vi "Agilent ENA Series Short Calibration.vi"() -> ()   [LabVIEW 2020]
doc: "Performs short calibration for port 1 and port 2.\n\nFor this VI you must set SHORT Port 1 and Port 2 on instrument."
uses:
  <instrlib>/Agilent ENA Series/Agilent ENA Series.lvlib
panel:
  in  "Reset? (T: Yes)":bool=TRUE
  in  "ID Query? (T: Yes)":bool=TRUE
  in  "VISA resource name":refnum<visa-resource-name>
  # "(c) 2005-2021 National Instruments.  ALL RIGHTS RESERVED."
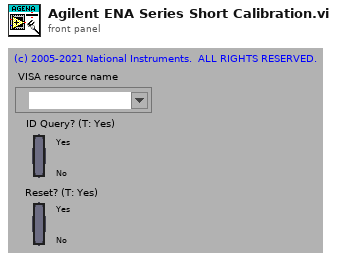
[diagram p1: front panel]
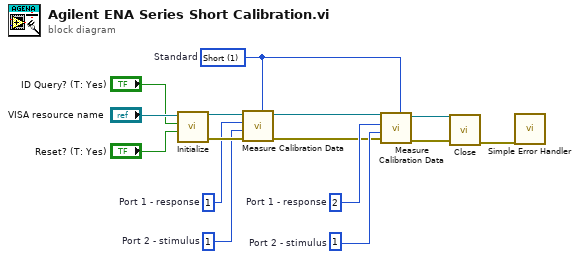
[diagram p0: block diagram]
diagram:
  w6 = 1  # Port 2 - stimulus
  w7 = 2  # Port 1 - response
  w9 = 1  # Port 2 - stimulus
  w10 = 1  # Port 1 - response
  w8 = u16 1 items=["Open", "Short", "Load", "Trhu", "Isolation"]  # Standard
  n1 = call <instrlib>:"Initialize.vi"("Reset? (T: Yes)"="Reset? (T: Yes)", "ID Query? (T: Yes)"="ID Query? (T: Yes)", "VISA resource name"="VISA resource name") -> ("error out"=w11:errorcluster, "VISA resource name out"=w12:refnum<visa-resource-name>)  [unwired: 7 in]
  n2 = call <instrlib>:"Measure Calibration Data.vi"("Standard (0: Open)"=w8, "error in (no error)"=w11, "Port 2 - stimulus (2)"=w9, "Port 1 - response (1)"=w10, "VISA resource name"=w12) -> ("error out"=w1:errorcluster, "VISA resource name out"=w2:refnum<visa-resource-name>)  [unwired: 5 in]
  n3 = call <instrlib>:"Measure Calibration Data.vi"("Standard (0: Open)"=w8, "error in (no error)"=w1, "Port 2 - stimulus (2)"=w6, "Port 1 - response (1)"=w7, "VISA resource name"=w2) -> ("error out"=w4:errorcluster, "VISA resource name out"=w5:refnum<visa-resource-name>)  [unwired: 5 in]
  n4 = call <instrlib>:"Close.vi"("error in (no error)"=w4, "VISA resource name"=w5) -> ("error out"=w3:errorcluster)  [unwired: 9 in]
  n5 = call <vilib>:"Simple Error Handler.vi"("error in (no error)"=w3) -> ()  [unwired: 4 in, 5 out]
